vi "data sample half.vi"(11 "배열":string[](array[string])) -> (3 "배열 2":string[](array[string]))   [LabVIEW 2015]
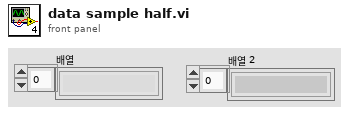
[diagram p1: front panel]
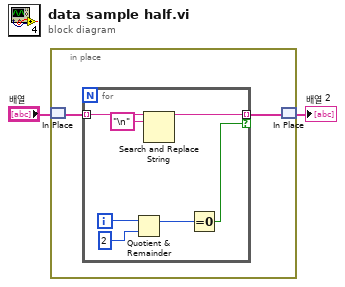
[diagram p0: block diagram]
diagram:
  n1 = in-place {
    n2 = in-place-match #1("배열") -> (w4:string[])
    n3 = for {
      tunnel: w4 -> [w7] mode=indexing
      tunnel: [w5] -> w3 mode=indexing if=w8
      i -> [w11]
      n4 = Quotient & Remainder(x=w11, y=2) -> (x-y*floor(x/y)=w9:i32)  [unwired: 1 out]
      n5 = Search and Replace String(input string=w7, search string="\n" ("검색 문자열")) -> (result string=w5:string)  [unwired: 6 in, 3 out]
      n6 = Equal To 0?(x=w9) -> (x = 0?=w8:bool)
    }
    n7 = in-place-match #1(w3) -> (→"배열 2":string[])
  }
